vi "Extractvalue.vi"(1 "Mesure":string, 2 "Chaîne":string) -> (0 "Value":dbl)   [LabVIEW 2018]
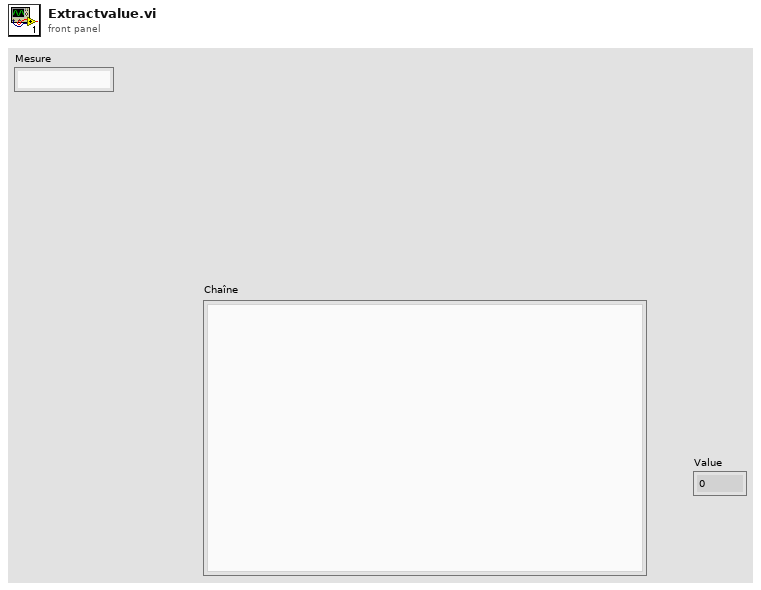
[diagram p1: front panel]
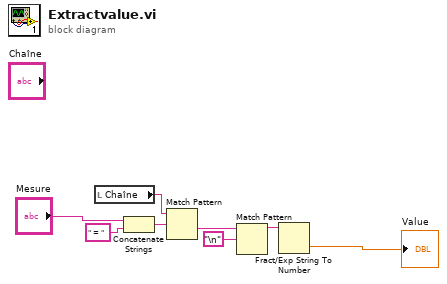
[diagram p0: block diagram]
diagram:
  n1 = local read "Chaîne"() -> (w8:string)
  n2 = Concatenate Strings("Mesure", " = " ("regular expression")) -> (w2:string)
  n3 = Match Pattern(string=w8, regular expression=w2) -> (after substring=w7:string)  [unwired: 1 in, 3 out]
  n4 = Match Pattern(string=w7, regular expression="\n") -> (before substring=w5:string)  [unwired: 1 in, 3 out]
  n5 = Fract/Exp String To Number(string=w5) -> (number=→"Value":dbl)  [unwired: 3 in, 1 out]
